vi "Current Position Write.vi"(4 "error in (no error)":errorcluster, 5 "Value":i32, 6 "Container State":T2, 7 "Display State In":T1) -> (0 "error out":errorcluster, 3 "Display State Out":T1)   [LabVIEW 2018, in "Vector Function Generator.xctl"]
doc: "Sets the location of the current position marker"
uses:
  Vector Function Generator.xctl
  <vilib>/_xctls/Container State.ctl
  Vector State.ctl
  <vilib>/_xctls/XControlSupport.lvlib
panel:
  # "Replace the Value Control below with a Control of desired type.\nDo not remove this Control or the others from the connector pane.\nDo not change the connector pane pattern.\nThe Value control should always be the third terminal from top on the input side in the connector pane."
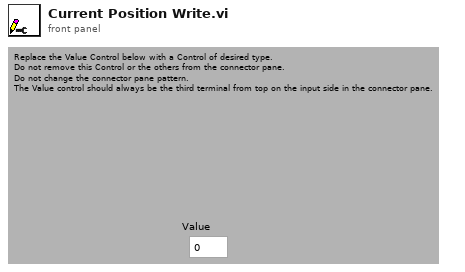
[diagram p1: front panel]
types:
  T1 = typedef "Vector Function Generator.xctl/Vector State.ctl" = cluster{"Current Position":i32, "Show Current Position":bool, "Mode (F=Polar)":bool, "digits":i32, "sf(F) or dp ?":bool, "Units":string}
  T2 = typedef "XControlSupport.lvlib/Container State.ctl" = cluster{"Indicator?":bool, "Run Mode?":bool, " Refnum":refnum<vi>}
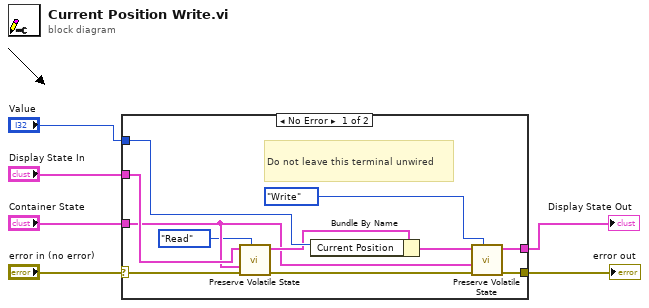
[diagram p0: block diagram]
diagram:
  n1 = case shown="No Error" "error in (no error)" {
    selector: "error in (no error)" -> [w16 w19]
    tunnel: "Value" -> [w17 _]
    tunnel: "Display State In" -> [w15 w18]
    tunnel: [w12 w18] -> w2
    tunnel: "Container State" -> [w8 _]
    tunnel: [w9 w19] -> w1
    frame No Error {
      # "Do not leave this terminal unwired"
      n2 = call "Preserve Volatile State.vi"("Operation In"=enum16{"Read", "Write", "Update From Data"}."Read" ("Operation"), "Error In (no Error) In"=w16, "Container State In"=w8, "Waveform State In"=w15) -> ("Error Out"=w11:errorcluster, "Waveform State Out"=w14:T1)  [unwired: 1 in, 5 out]
      n3 = Bundle By Name(cluster=w14, "Current Position"=w17) -> (w13:T1)
      n4 = call "Preserve Volatile State.vi"("Operation In"=enum16{"Read", "Write"}."Write" ("Operation"), "Error In (no Error) In"=w11, "Container State In"=w8, "Waveform State In"=w13) -> ("Error Out"=w9:errorcluster, "Waveform State Out"=w12:T1)  [unwired: 1 in, 5 out]
    }
    frame Error {
    }
  }
  "error out" <- w1
  "Display State Out" <- w2
